vi "Generate XY Matrix.vi"(1 "XY":cluster{"X":i32, "Y":i32}) -> (0 "XY Matrix":T1)   [LabVIEW 2019, in "Referential.lvclass"]
uses:
  Referential.lvclass
  <vilib>/Analysis/Matrix/Datatypes/RealMatrix.ctl
  <vilib>/Analysis/Matrix/NI_Matrix.lvlib
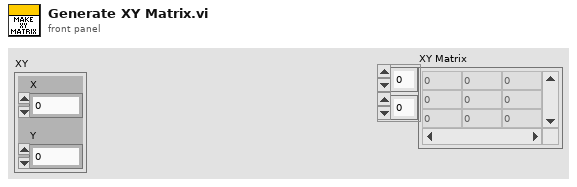
[diagram p1: front panel]
types:
  T1 = typedef "NI_Matrix.lvlib/RealMatrix.ctl" = dbl[][]
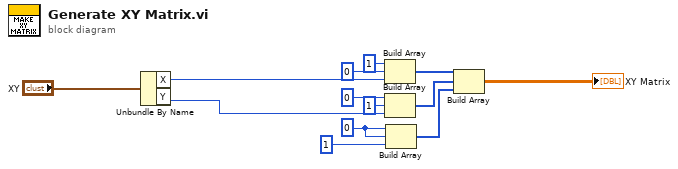
[diagram p0: block diagram]
diagram:
  w12 = 0 ("element")
  n1 = Unbundle By Name("XY") -> ("X"=w3:i32, "Y"=w2:i32)
  n2 = Build Array(1 ("element"), 0 ("element"), w3) -> (w7:i32[])
  n3 = Build Array(0 ("element"), 1 ("element"), w2) -> (w6:i32[])
  n4 = Build Array(w12, w12, 1 ("element")) -> (w5:i32[])
  n5 = Build Array(w7, w6, w5) -> (→"XY Matrix":T1)
